vi "Disconnect.vi"(8 "error in (no error)":errorcluster, 11 "Statnett C37.118 DLL in":refnum<class "Statnett C37.118 DLL.lvclass">) -> (0 "error out":errorcluster, 3 "Statnett C37.118 DLL out":refnum<class "Statnett C37.118 DLL.lvclass">)   [LabVIEW 2013, in "PMU Recorder Light.lvlib" / "Statnett C37.118 DLL.lvclass"]
uses:
  Statnett C37.118 DLL.lvclass
  Statnett C37.118 DLL.lvclass/Statnett C37.118 DLL.ctl
  c37118-dll/labview/C37118-DLL.lvlib
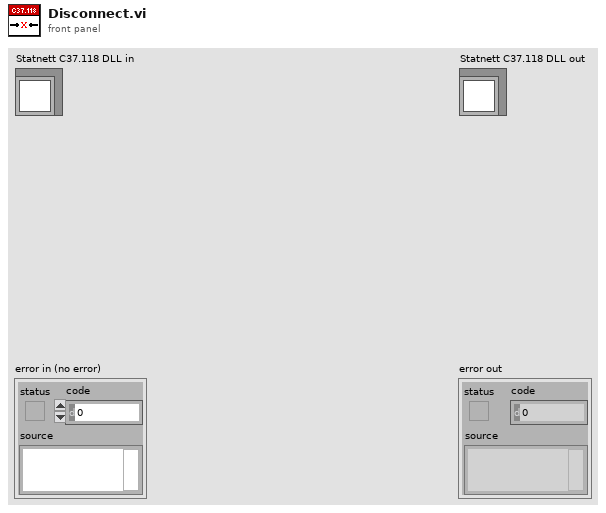
[diagram p1: front panel]
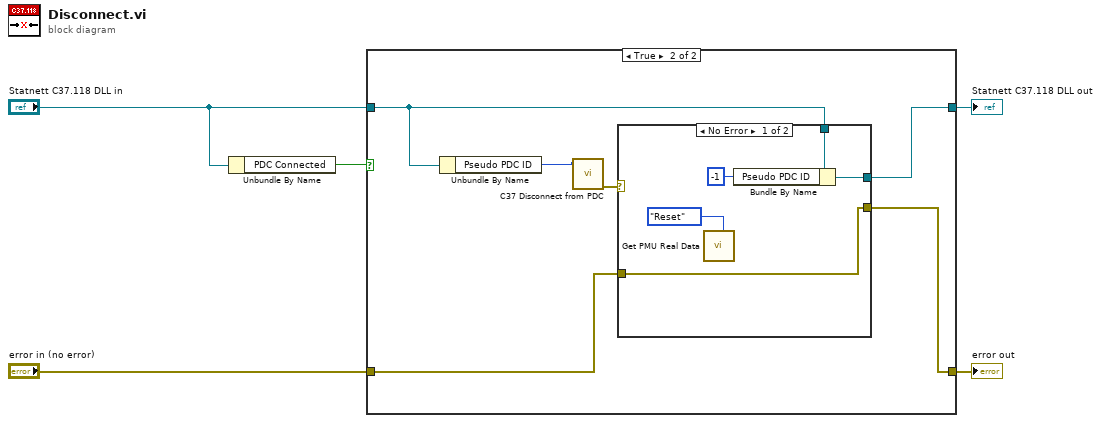
[diagram p0: block diagram]
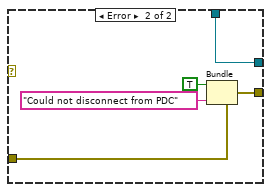
[diagram p3: hidden frame]
diagram:
  n1 = Unbundle By Name("Statnett C37.118 DLL in") -> ("PDC Connected"=w1:bool)
  n2 = case shown="True" w1 {
    tunnel: "error in (no error)" -> [w6 w13]
    tunnel: [w6 w12] -> w4
    tunnel: "Statnett C37.118 DLL in" -> [w7 w10]
    tunnel: [w7 w11] -> w3
    frame False {
    }
    frame True {
      n3 = Unbundle By Name(w10) -> ("Pseudo PDC ID"=w9:i32)
      n4 = call "C37 Disconnect from PDC.vi"("Pseudo PDC ID"=w9) -> ("error out"=w8:errorcluster)  [unwired: 10 in]
      n5 = case shown="No Error" w8 {
        tunnel: w13 -> [w18 w23]
        tunnel: [w18 w20] -> w12
        tunnel: w10 -> [w17 w19]
        tunnel: [w15 w19] -> w11
        frame No Error {
          n6 = call "Get PMU Real Data.vi"("Action"=enum16{"Initialize", "Read", "Reset"}."Reset") -> ()  [unwired: 8 in, 3 out]
          n7 = Bundle By Name(cluster=w17, "Pseudo PDC ID"=-1) -> (w15:refnum<class "Statnett C37.118 DLL.lvclass">)
        }
        frame Error {
          n8 = Bundle(cluster=w23, "status"=TRUE, "source"="Could not disconnect from PDC") -> (w20:errorcluster)  [unwired: 1 in]
        }
      }
    }
  }
  "error out" <- w4
  "Statnett C37.118 DLL out" <- w3
